vi "_01_FGV Structure (in depth).vi"() -> ()   [LabVIEW 2020]
panel:
  in  "Action's":enum16{"Write Data", "Read Data"}(ring)
  out "Output":dbl
  in  "Input":dbl
  out "error out":errorcluster
  in  "error in (no error)":errorcluster
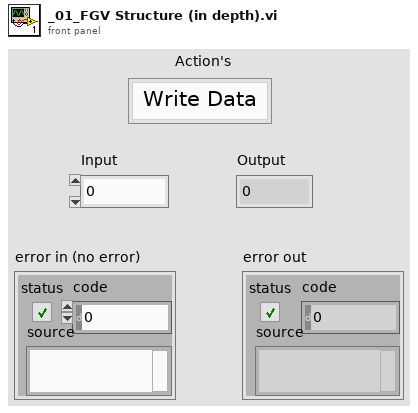
[diagram p1: front panel]
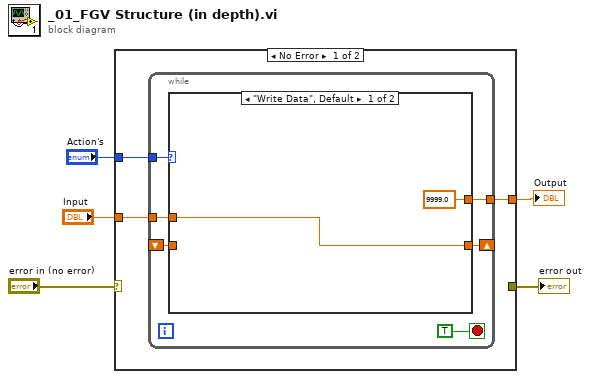
[diagram p0: block diagram]
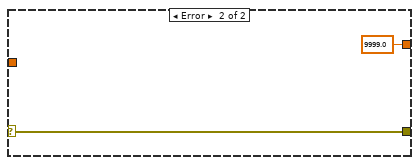
[diagram p3: hidden frame]
diagram:
  n1 = case shown="No Error" "error in (no error)" {
    selector: "error in (no error)" -> [_ w19]
    tunnel: [_ w19] -> w4
    tunnel: "Action's" -> [w8 _]
    tunnel: "Input" -> [w7 _]
    tunnel: [w6 9999.0 ("Numeric")] -> w1
    frame No Error {
      n2 = while {
        tunnel: w8 -> [w14]
        shift-right: [w10] -> _
        shift-left: _ -> [w12]
        tunnel: w7 -> [w13]
        tunnel: [w11] -> w6
        stop <- TRUE stop-if-true
        n3 = case shown="\"Write Data\", Default" w14 {
          tunnel: w13 -> [w16 _]
          tunnel: w12 -> [_ w17]
          tunnel: [w16 w17] -> w10
          tunnel: [9999.0 ("Numeric") w17] -> w11
          frame "Write Data", Default {
          }
          frame "Read Data" {
          }
        }
      }
    }
    frame Error {
    }
  }
  "Output" <- w1
  "error out" <- w4
